vi "Create SV channels.vi"(8 "error in":errorcluster, 10 "Variable List":refnum<class "Channel.lvclass">[](array[class]), 11 "Custom Device in":T1 format="%.0x") -> (0 "error out":errorcluster, 3 "Device Ref out":T1 format="%.0x")   [LabVIEW 2021, in "Shared Variables CD 2.0 Configuration.lvlib" / "ChannelVS.lvclass"]
uses:
  ChannelVS.lvclass
  ChannelVS.lvclass/ChannelVS.ctl
  <vilib>/NI VeriStand/Custom Device API/Custom Device API.lvlib
  <vilib>/NI VeriStand/Custom Device API/Custom Device Channel Type.ctl
  <vilib>/NI VeriStand/Custom Device API/Custom Device Channel.ctl
  Shared/Shared Variables CD 2.0 GUID Lookup.vi
  Shared/SV Global.vi
  <vilib>/NI VeriStand/Custom Device API/Custom Device Item Ref.ctl
  OneDrive - NI/Documents/GitHub/Shared-Variable-Custom-Device-2.0/Modules/Channel.lvlibp/Channel.lvclass
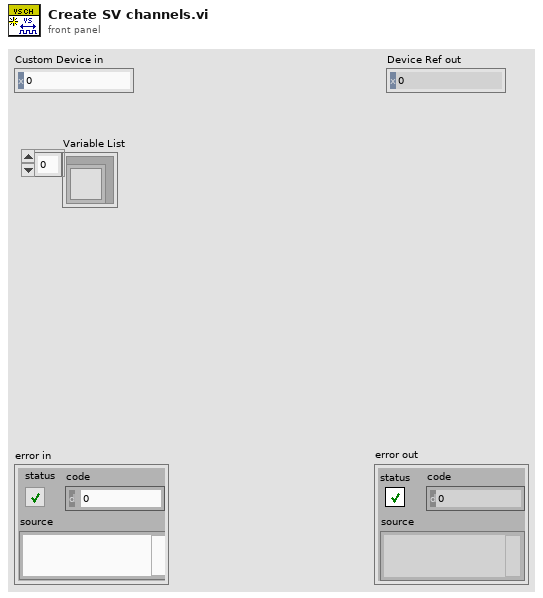
[diagram p1: front panel]
types:
  T1 = typedef "Custom Device API.lvlib/Custom Device Item Ref.ctl" = u64
  T2 = typedef "Custom Device API.lvlib/Custom Device Channel.ctl" = cluster{"Type":T3, "Units":string, "Default Value":dbl, "Faultable":bool, "Scalable":bool}
  T3 = typedef "Custom Device API.lvlib/Custom Device Channel Type.ctl" = enum16{"Input", "Output"}
  T4 = typedef "Channel.lvlibp/NI_Data Type.lvlib/Data Type.ctl" = enum8{"Invalid Type", "Void", "I8", "I16", "I32", "I64", "U8", "U16", "U32", "U64", "Single Float", "Double Float", "Extended Float", "Single Complex", "Double Complex", "Extended Complex", "Enum U8", "Enum U16", "Enum U32", "Enum U64", "Single Float With Unit", "Double Float With Unit", "Extended Float With Unit", "Single Complex with Unit", "Double Complex with Unit", "Extended Complex with Unit", "Boolean", "String", "Path", "Picture", "Tag", "Array", "Cluster", "Variant", "LV Variant", "Waveform", "Timestamp", "Digital Waveform", "Digital Data", "ExpressData", "Refnum", "External Data", "VI", "Poly VI", "LabVIEW Class Instance", "Fixed Point", "Set Collection", "Map Collection"}
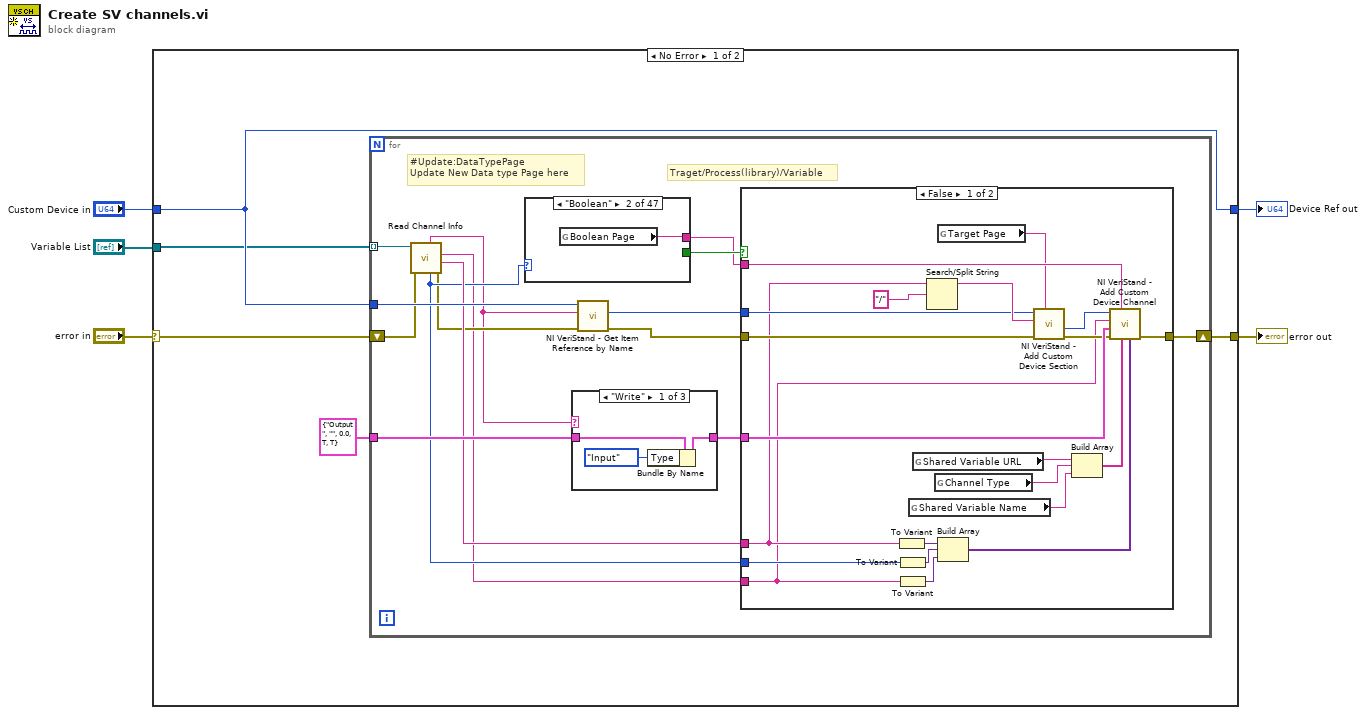
[diagram p0: block diagram]
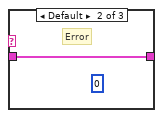
[diagram p2: hidden frame]
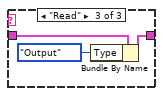
[diagram p3: hidden frame]
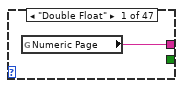
[diagram p4: hidden frame]
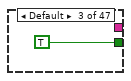
[diagram p5: hidden frame]
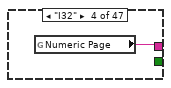
[diagram p6: hidden frame]
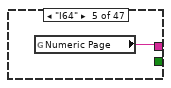
[diagram p7: hidden frame]
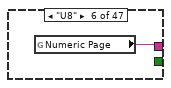
[diagram p8: hidden frame]
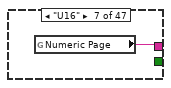
[diagram p9: hidden frame]
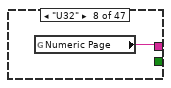
[diagram p10: hidden frame]
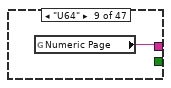
[diagram p11: hidden frame]
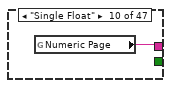
[diagram p12: hidden frame]
diagram:
  n1 = case shown="No Error" "error in" {
    selector: "error in" -> [w9 w68]
    tunnel: "Custom Device in" -> [w8 w67]
    tunnel: [w10 w68] -> w4
    tunnel: "Variable List" -> [w7 _]
    tunnel: [w8 w67] -> w1
    frame No Error {
      n2 = for {
        shift-right: [w25] -> w10
        shift-left: w9 -> [w21]
        tunnel: w8 -> [w24]
        tunnel: w7 -> [w23] mode=indexing
        tunnel: T2 {"Type"=enum."Output", "Units"="", "Default Value"=0.0, "Faultable"=TRUE, "Scalable"=TRUE} ("Channel") -> [w22]
        # "#Update:DataTypePage\nUpdate New Data type Page here"
        # "Traget/Process(library)/Variable"
        n3 = call "Read Channel Info.vi"("error in (no error)"=w21, "Channel in"=w23) -> ("error out"=w13:errorcluster, "URL"=w18:string, "Name"=w12:string, "DataType"=w17:T4, "Read or Write"=w11:string)  [unwired: 4 in, 1 out]
        n4 = case shown="\"Boolean\"" w17 {
          tunnel: [_ _ TRUE _ _ _ _ _ _ _ _ _ _ _ _ _ _ _ _ _ _ _ _ _ _ _ _ _ _ _ _ _ _ _ _ _ _ _ _ _ _ _ _ _ _ _ _] -> w20
          tunnel: [w33 w34 _ w36 w37 w38 w39 w40 w41 w42 _ _ _ _ _ _ _ _ _ _ _ _ _ _ _ _ _ _ _ _ _ _ _ _ _ _ _ _ _ _ _ _ _ w43 w44 _ _] -> w19
          frame "Double Float" {
            n5 = global read "Shared Variables CD 2.0 GUID Lookup.vi" "Numeric Page"() -> (w33:string)
          }
          frame "Boolean" {
            n6 = global read "Shared Variables CD 2.0 GUID Lookup.vi" "Boolean Page"() -> (w34:string)
          }
          frame Default {
          }
          frame "I32" {
            n7 = global read "Shared Variables CD 2.0 GUID Lookup.vi" "Numeric Page"() -> (w36:string)
          }
          frame "I64" {
            n8 = global read "Shared Variables CD 2.0 GUID Lookup.vi" "Numeric Page"() -> (w37:string)
          }
          frame "U8" {
            n9 = global read "Shared Variables CD 2.0 GUID Lookup.vi" "Numeric Page"() -> (w38:string)
          }
          frame "U16" {
            n10 = global read "Shared Variables CD 2.0 GUID Lookup.vi" "Numeric Page"() -> (w39:string)
          }
          frame "U32" {
            n11 = global read "Shared Variables CD 2.0 GUID Lookup.vi" "Numeric Page"() -> (w40:string)
          }
          frame "U64" {
            n12 = global read "Shared Variables CD 2.0 GUID Lookup.vi" "Numeric Page"() -> (w41:string)
          }
          frame "Single Float" {
            n13 = global read "Shared Variables CD 2.0 GUID Lookup.vi" "Numeric Page"() -> (w42:string)
          }
          frame "Extended Float" {
          }
          frame "Single Complex" {
          }
          frame "Double Complex" {
          }
          frame "Extended Complex" {
          }
          frame "Enum U8" {
          }
          frame "Enum U16" {
          }
          frame "Enum U32" {
          }
          frame "Enum U64" {
          }
          frame "Single Float With Unit" {
          }
          frame "Double Float With Unit" {
          }
          frame "Extended Float With Unit" {
          }
          frame "Single Complex with Unit" {
          }
          frame "Double Complex with Unit" {
          }
          frame "Extended Complex with Unit" {
          }
          frame "String" {
          }
          frame "Path" {
          }
          frame "Picture" {
          }
          frame "Tag" {
          }
          frame "Array" {
          }
          frame "Cluster" {
          }
          frame "Variant" {
          }
          frame "LV Variant" {
          }
          frame "Waveform" {
          }
          frame "Timestamp" {
          }
          frame "Digital Waveform" {
          }
          frame "Digital Data" {
          }
          frame "ExpressData" {
          }
          frame "Refnum" {
          }
          frame "External Data" {
          }
          frame "VI" {
          }
          frame "Poly VI" {
          }
          frame "LabVIEW Class Instance" {
          }
          frame "Fixed Point" {
          }
          frame "I16" {
            n14 = global read "Shared Variables CD 2.0 GUID Lookup.vi" "Numeric Page"() -> (w43:string)
          }
          frame "I8" {
            n15 = global read "Shared Variables CD 2.0 GUID Lookup.vi" "Numeric Page"() -> (w44:string)
          }
          frame "Void" {
          }
          frame "Invalid Type" {
          }
        }
        n16 = case shown="\"Write\"" w11 {
          tunnel: w22 -> [w28 w29 w32]
          tunnel: [w26 w29 w30] -> w16
          frame "Write" {
            n17 = Bundle By Name(cluster=w28, "Type"=Custom_Device_Channel_Type."Input") -> (w26:T2)
          }
          frame Default {
            (unwired) T1 0 ("Section Ptr")
            # "Error"
          }
          frame "Read" {
            n18 = Bundle By Name(cluster=w32, "Type"=Custom_Device_Channel_Type."Output") -> (w30:T2)
          }
        }
        n19 = call <vilib>:"NI VeriStand - Get Item Reference by Name.vi"("error in (no error)"=w13, "Item Name"=w11, "Parent Ref in"=w24) -> ("error out"=w14:errorcluster, "Item Ref"=w15:T1)  [unwired: 5 in, 2 out]
        n20 = case shown="False" w20 {
          tunnel: w19 -> [w65 _]
          tunnel: w16 -> [w64 _]
          tunnel: [w58 w66] -> w25
          tunnel: w17 -> [w49 _]
          tunnel: w18 -> [w46 _]
          tunnel: w12 -> [w45 _]
          tunnel: w15 -> [w48 _]
          tunnel: w14 -> [w47 w66]
          frame False {
            n21 = To Variant(anything=w46) -> (Variant=w62:variant)
            n22 = To Variant(anything=w49) -> (Variant=w61:variant)
            n23 = To Variant(anything=w45) -> (Variant=w59:variant)
            n24 = global read "SV Global.vi" "Shared Variable Name"() -> (w51:string)
            n25 = global read "SV Global.vi" "Shared Variable URL"() -> (w52:string)
            n26 = Search/Split String(string=w46, search string/char (-)="/") -> (substring before match=w54:string)  [unwired: 1 in, 2 out]
            n27 = global read "SV Global.vi" "Channel Type"() -> (w50:string)
            n28 = global read "Shared Variables CD 2.0 GUID Lookup.vi" "Target Page"() -> (w55:string)
            n29 = Build Array(w62, w61, w59) -> (w60:variant[])
            n30 = call <vilib>:"NI VeriStand - Add Custom Device Section.vi"("GUID (Default Section)"=w55, "error in (no error)"=w47, "Section Name"=w54, "Parent Ref in"=w48) -> ("error out"=w56:errorcluster, "Section Ptr"=w57:T1)  [unwired: 4 in, 2 out]
            n31 = Build Array(w52, w50, w51) -> (w63:string[])
            n32 = call <vilib>:"NI VeriStand - Add Custom Device Channel.vi"("Property Values"=w60, "Property names"=w63, "GUID (Default Channel)"=w65, "error in (no error)"=w56, "Channel"=w64, "Channel Name"=w45, "Parent Ref in"=w57) -> ("error out"=w58:errorcluster)  [unwired: 1 in, 3 out]
          }
          frame True {
          }
        }
      }
    }
    frame Error {
    }
  }
  "error out" <- w4
  "Device Ref out" <- w1
